vi "9-WriteAccessTest.vi"() -> ()   [LabVIEW 2016, in "TestVIs.lvlib"]
uses:
  TestVIs.lvlib
panel:
  out "Array 2":cluster{"Name":string, "permissions":i16}[](array[cluster])
  out "Array":string[](array[string])
  out "Name":string
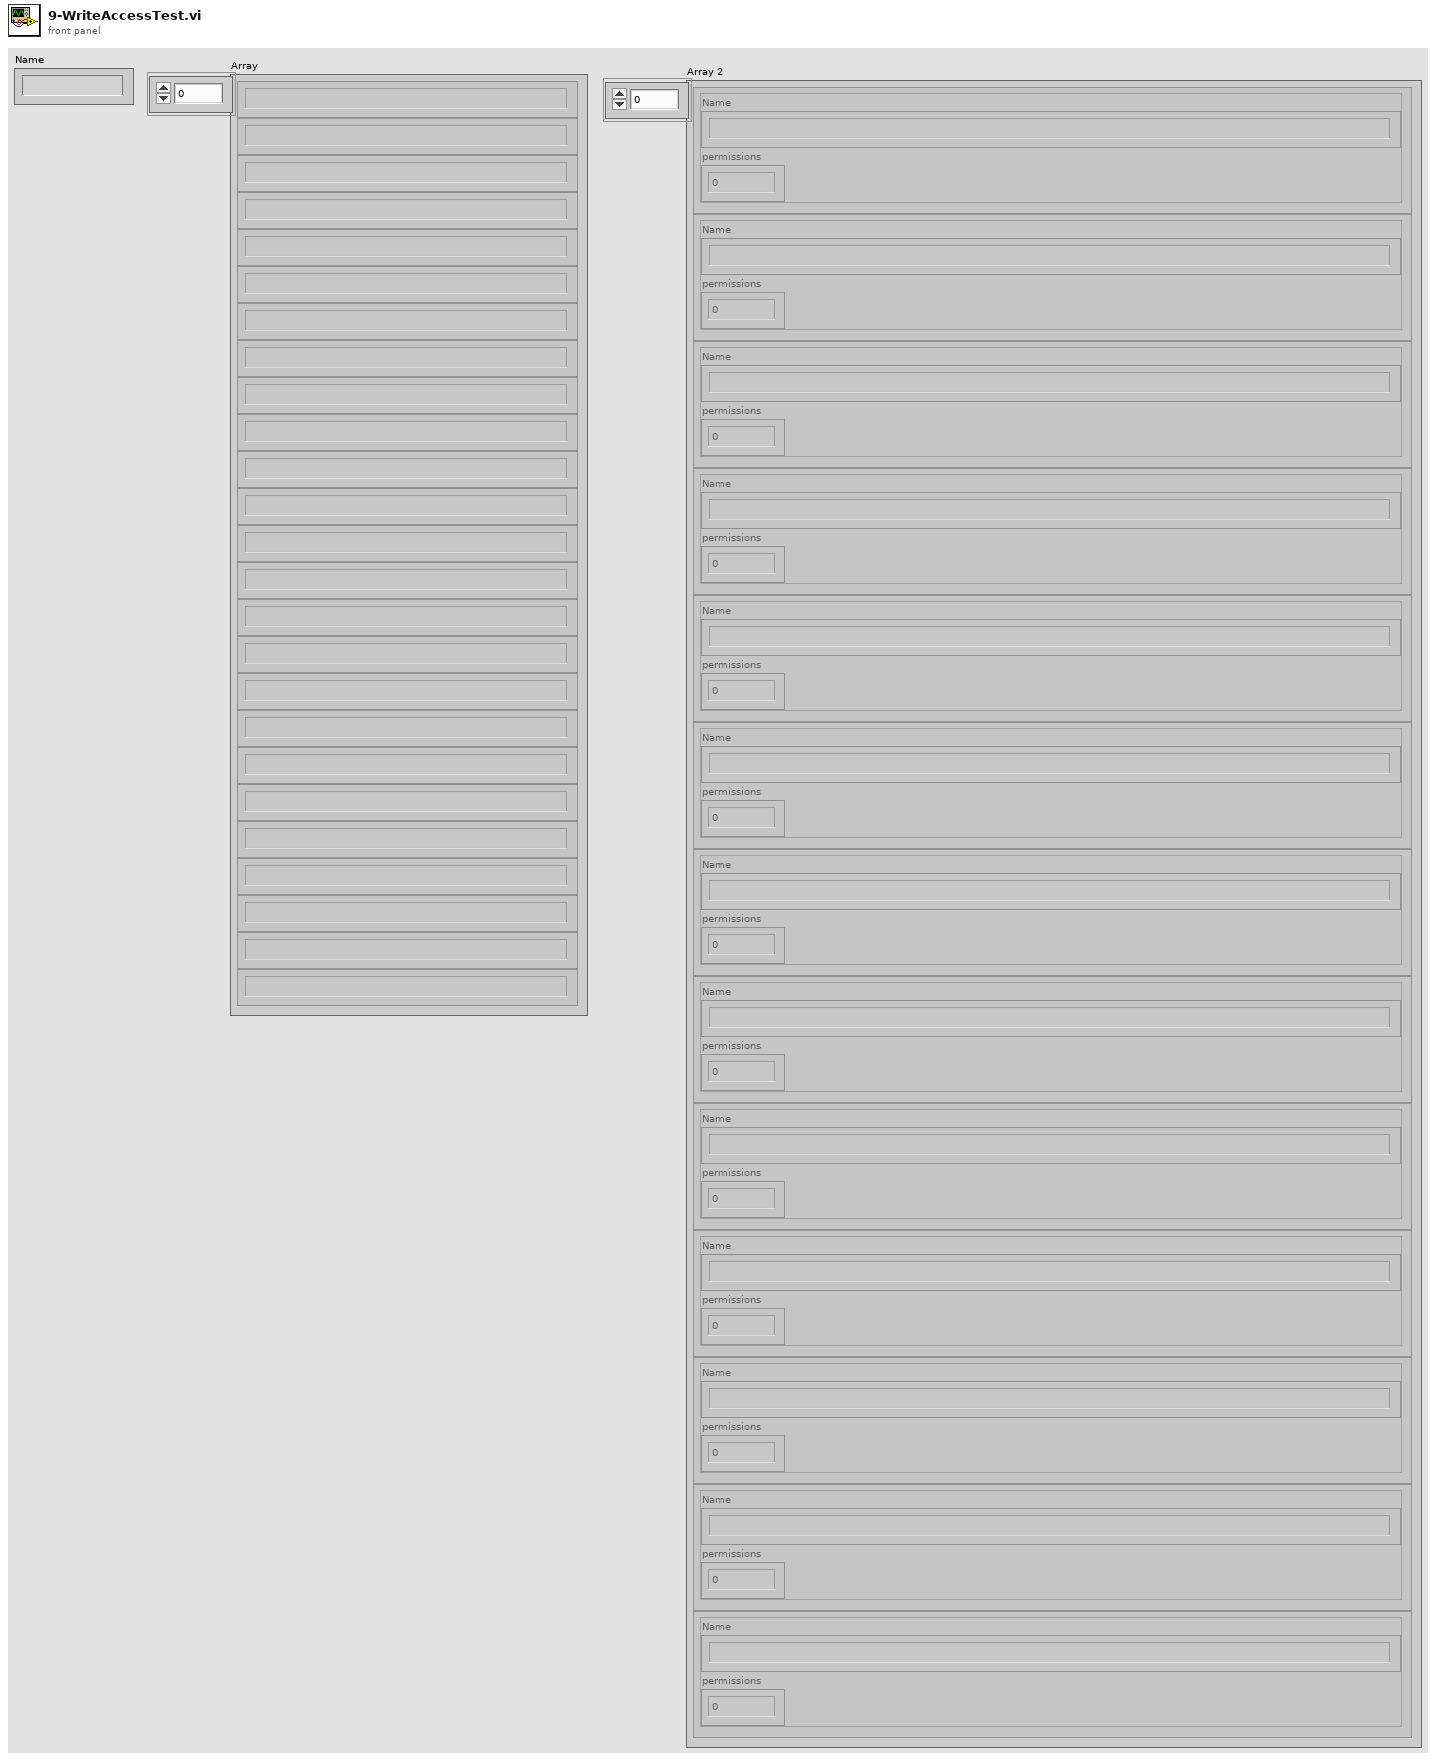
[diagram p1: front panel]
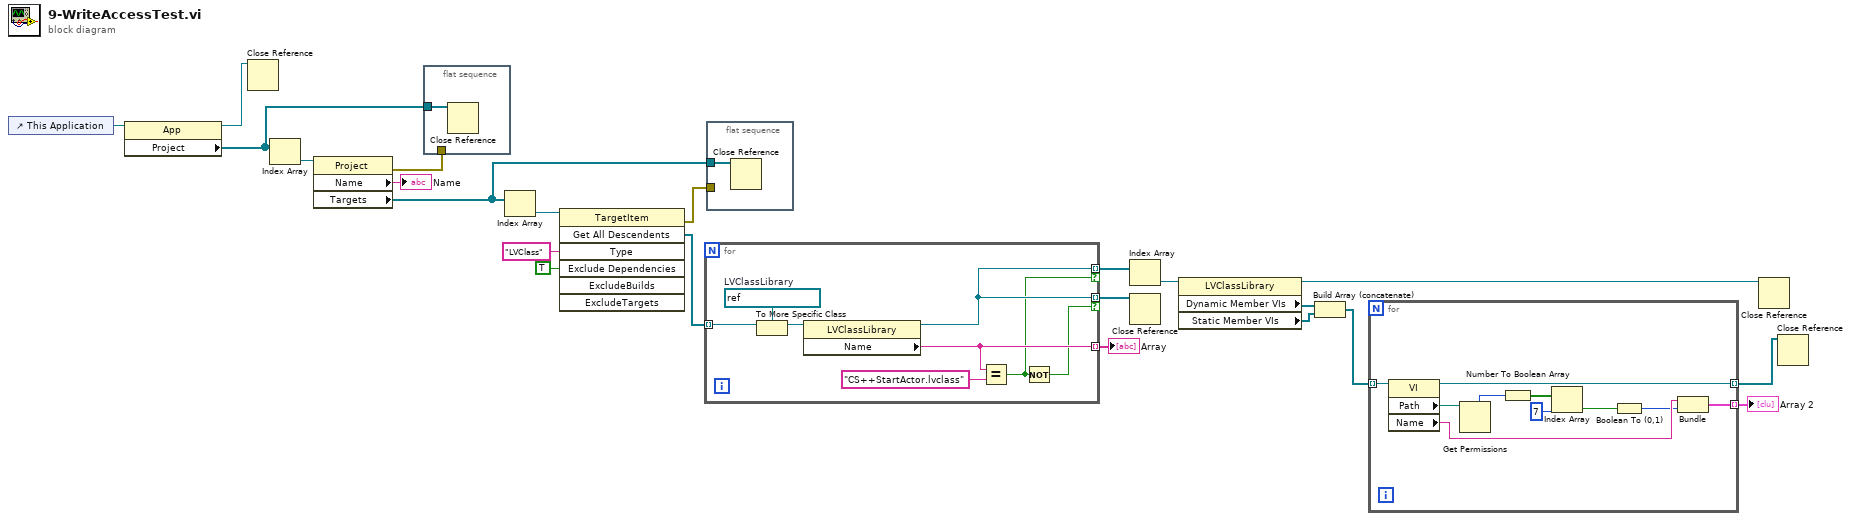
[diagram p0: block diagram]
diagram:
  n1 = control-ref of="This Application"() -> (w22:refnum<vi>)
  n2 = property class="App"(reference=w22) -> (reference out=w19:refnum<vi>, "Project"=w18:refnum<vi>[])  [unwired: 1 in, 1 out]
  n3 = Close Reference(reference=w19) -> ()  [unwired: 1 in, 1 out]
  n4 = Index Array(array=w18) -> (element=w21:refnum<vi>)  [unwired: 1 in]
  n5 = property class="Project"(reference=w21) -> (error out=w17:errorcluster, "Name"=→"Name":string, "Targets"=w16:refnum<vi>[])  [unwired: 1 in, 1 out]
  n6 = flat-sequence {
    tunnel: w18 -> [w23]
    tunnel: w17 -> [_]
    frame #0 {
      n7 = Close Reference(reference=w23) -> ()  [unwired: 1 in, 1 out]
    }
  }
  n8 = Index Array(array=w16) -> (element=w13:refnum<vi>)  [unwired: 1 in]
  n9 = invoke class="TargetItem" method="Get All Descendents"(reference=w13, "Type"="LVClass", "Exclude Dependencies"=TRUE ("ExcludeDependencies")) -> (error out=w12:errorcluster, "All Descendents"=w11:refnum<vi>[])  [unwired: 4 in, 5 out]
  n10 = for {
    tunnel: w11 -> [w30] mode=indexing
    tunnel: [w28] -> w10 mode=indexing
    tunnel: [w25] -> w9 mode=indexing if=w26
    tunnel: [w25] -> w8 mode=indexing if=w24
    w31 = refnum<vi> refnum  # LVClassLibrary
    n11 = To More Specific Class(target class=w31, reference=w30) -> (specific class reference=w29:refnum<vi>)  [unwired: 1 in, 1 out]
    n12 = property class="LVClassLibrary"(reference=w29) -> (reference out=w25:refnum<vi>, "Name"=w28:string)  [unwired: 1 in, 1 out]
    n13 = Equal?(x=w28, y="CS++StartActor.lvclass") -> (x = y?=w24:bool)
    n14 = Not(x=w24) -> (.not. x?=w26:bool)
  }
  "Array" <- w10
  n15 = flat-sequence {
    tunnel: w16 -> [w32]
    tunnel: w12 -> [_]
    frame #0 {
      n16 = Close Reference(reference=w32) -> ()  [unwired: 1 in, 1 out]
    }
  }
  n17 = Index Array(array=w8) -> (element=w7:refnum<vi>)  [unwired: 1 in]
  n18 = Close Reference(reference=w9) -> ()  [unwired: 1 in, 1 out]
  n19 = property class="LVClassLibrary"(reference=w7) -> (reference out=w6:refnum<vi>, "Dynamic Member VIs"=w5:refnum<vi>[], "Static Member VIs"=w4:refnum<vi>[])  [unwired: 1 in, 1 out]
  n20 = Build Array (concatenate)(w5, w4) -> (w3:refnum<vi>[])
  n21 = for {
    tunnel: w3 -> [w42] mode=indexing
    tunnel: [w40] -> w2 mode=indexing
    tunnel: [w38] -> w1 mode=indexing
    n22 = property class="VI"(reference=w42) -> (reference out=w40:refnum<vi>, "Path"=w41:path, "Name"=w39:string)  [unwired: 1 in, 1 out]
    n23 = Get Permissions(11:w41) -> (5:w37:i16)  [unwired: 1 in, 4 out]
    n24 = Number To Boolean Array(number=w37) -> (Boolean array=w36:bool[])
    n25 = Index Array(array=w36, index=7) -> (element=w34:bool)
    n26 = Boolean To (0,1)(Boolean=w34) -> (0, 1=w33:i16)
    n27 = Bundle("Name"=w39, w33) -> (w38:cluster{"Name":string, i16})  [unwired: 1 in]
  }
  "Array 2" <- w1
  n28 = Close Reference(reference=w6) -> ()  [unwired: 1 in, 1 out]
  n29 = Close Reference(reference=w2) -> ()  [unwired: 1 in, 1 out]
